vi "AddSharedVariableToLibrary.vi"(6 "Variable Type (Network-Published)":T1(ring)=enum."Network-Published", 8 "error in (no error)":errorcluster, 9 "Variable Data Type (Double)":variant=variant(dbl 0.0), 10 "Variable Name":string, 11 "Library Reference In":refnum<vi>) -> (0 "error out":errorcluster, 2 "Variable Reference Out":refnum<vi>, 3 "Library Reference Out":refnum<vi>)   [LabVIEW 2020]
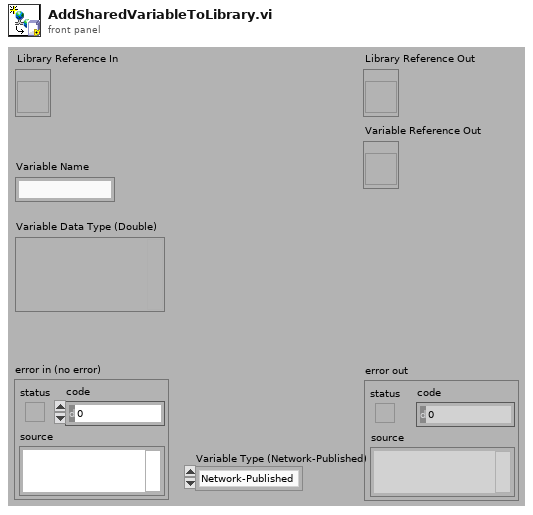
[diagram p1: front panel]
types:
  T1 = enum16{"Single-Process", "Network-Published", "Time-Triggered"}
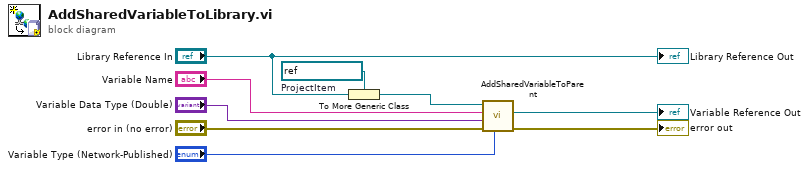
[diagram p0: block diagram]
diagram:
  w9 = refnum<vi> refnum  # ProjectItem
  n1 = To More Generic Class(target class=w9, reference="Library Reference In") -> (generic class reference=w8:refnum<vi>)
  n2 = call <vilib>:"AddSharedVariableToParent.vi"("Variable Type (Network-Published)"="Variable Type (Network-Published)", "error in (no error)"="error in (no error)", "Variable Data Type (Double)"="Variable Data Type (Double)", "Variable Name"="Variable Name", "Library Reference In"=w8) -> ("error out"=→"error out":errorcluster, "Variable Reference Out"=→"Variable Reference Out":refnum<vi>)  [unwired: 4 in, 1 out]
  "Library Reference Out" <- "Library Reference In"
